vi "FindBandwidth.vi"() -> ()   [LabVIEW 2022 SP3]
doc: "6/7/11- It doesnt really work."
uses:
  <vilib>/Analysis/baseanly.llb/Mean (DBL).vi
  <vilib>/Utility/file.llb/Read Delimited Spreadsheet (DBL).vi
  <vilib>/Analysis/NI_AALBase.lvlib
panel:
  in  "Define BW?":bool
  in  "non dB data?":bool=TRUE
  out "Array 2":T1(array[cluster]) {"bandwidth" format="%.2f"; "upper band freq" format="%.2f"; "lower band freq" format="%.2f"; "center freq" format="%.2f"; "max freq (dB)" format="%.2f"; "max f" format="%.2f"}
  out "DOF":cluster{dbl[], sgl[]}(graph)
  out "L BW":cluster{dbl[], dbl[]}(graph)
  in  "f cut off MHz":dbl=100.0
  out "Array":dbl[][](array[numeric])
  in  "file ext":string="*.txt"
  in  "Use Selected Files":bool
  in  "Listbox":i32[](listbox)
  in  "Choose Directory":path
  in  "Save path":path
  in  "Save?":bool
  out "XY Graph":cluster{"all rows":dbl[], "all rows":dbl[]}[](graph)
  in  "Save spectrum only":bool
  in  "dB width pt":dbl=-6.0 format="%.2f"
  # "max f"
  # "max f dB"
  # "fc 15 dB"
  # "BW 15db"
  # "fc 6 db"
  # "BW 6dB"
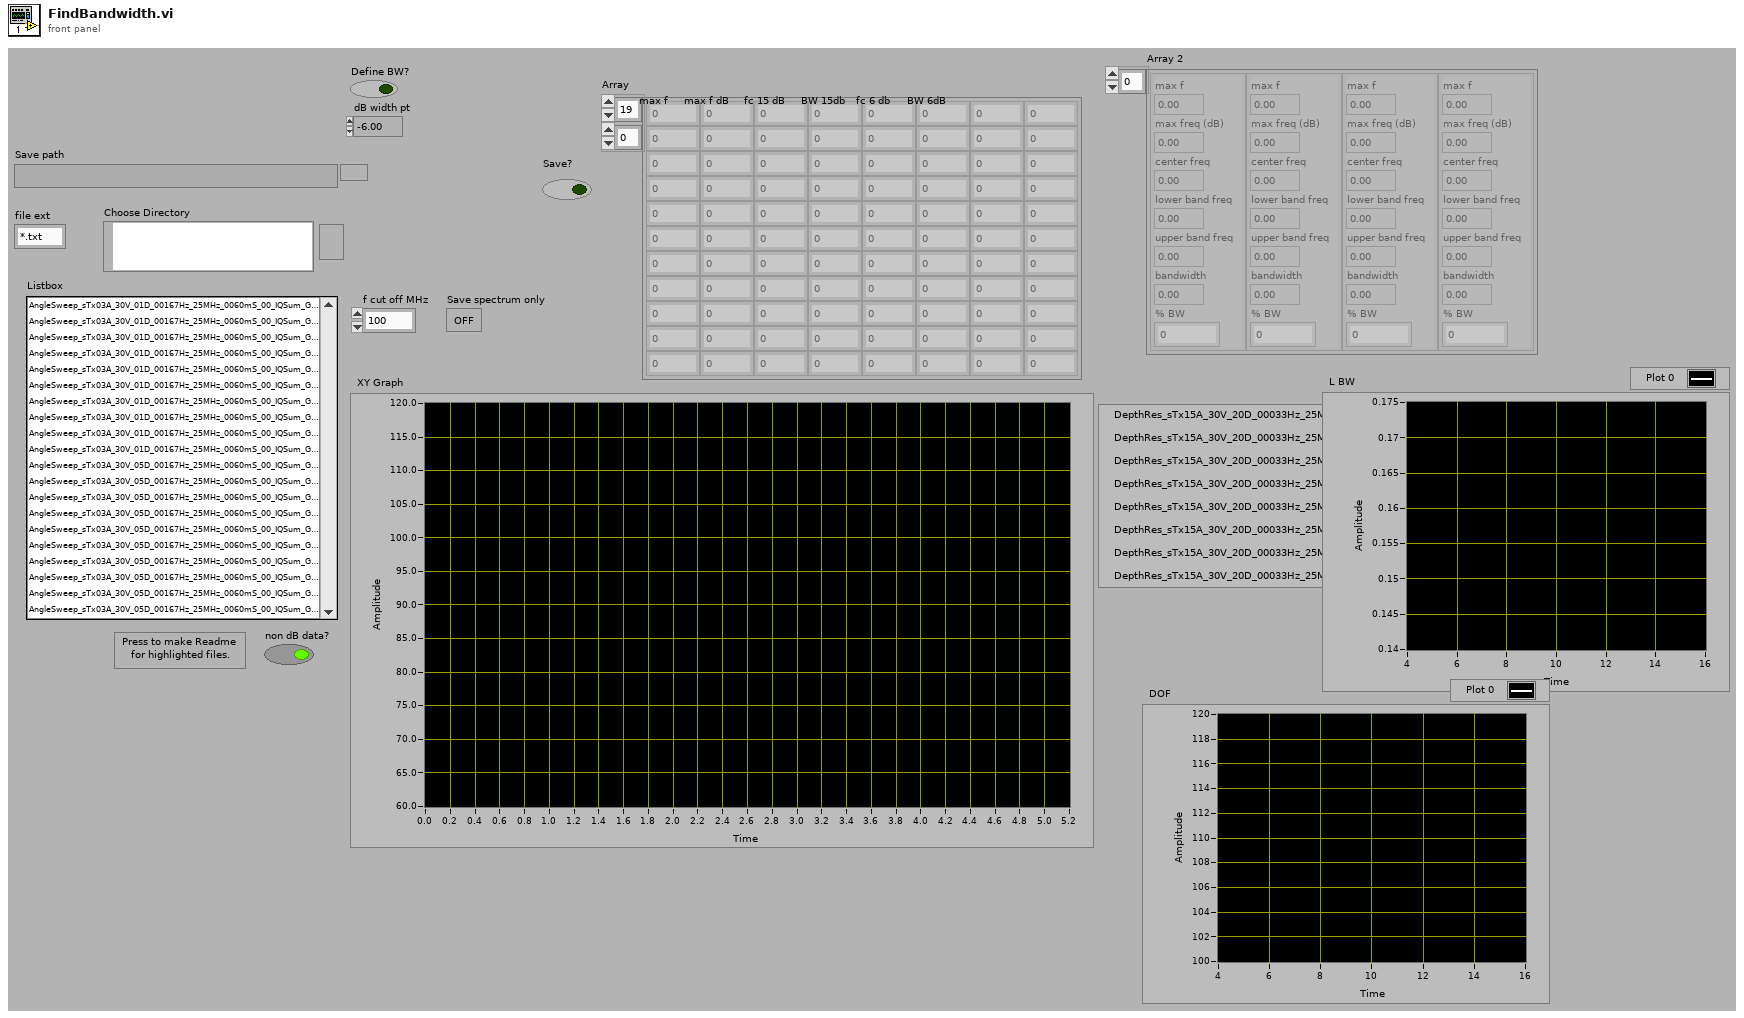
[diagram p1: front panel]
types:
  T1 = cluster{"max f":sgl, "max freq (dB)":sgl, "center freq":sgl, "lower band freq":sgl, "upper band freq":sgl, "bandwidth":sgl, "% BW":dbl}[]
  T2 = cluster{"max f":sgl, "max freq (dB)":sgl, "center freq":sgl, "lower band freq":sgl, "upper band freq":sgl, "bandwidth":sgl, "% BW":dbl}
  T3 = enum16{"open", "replace", "create", "open or create", "replace or create", "replace or create with confirmation"}
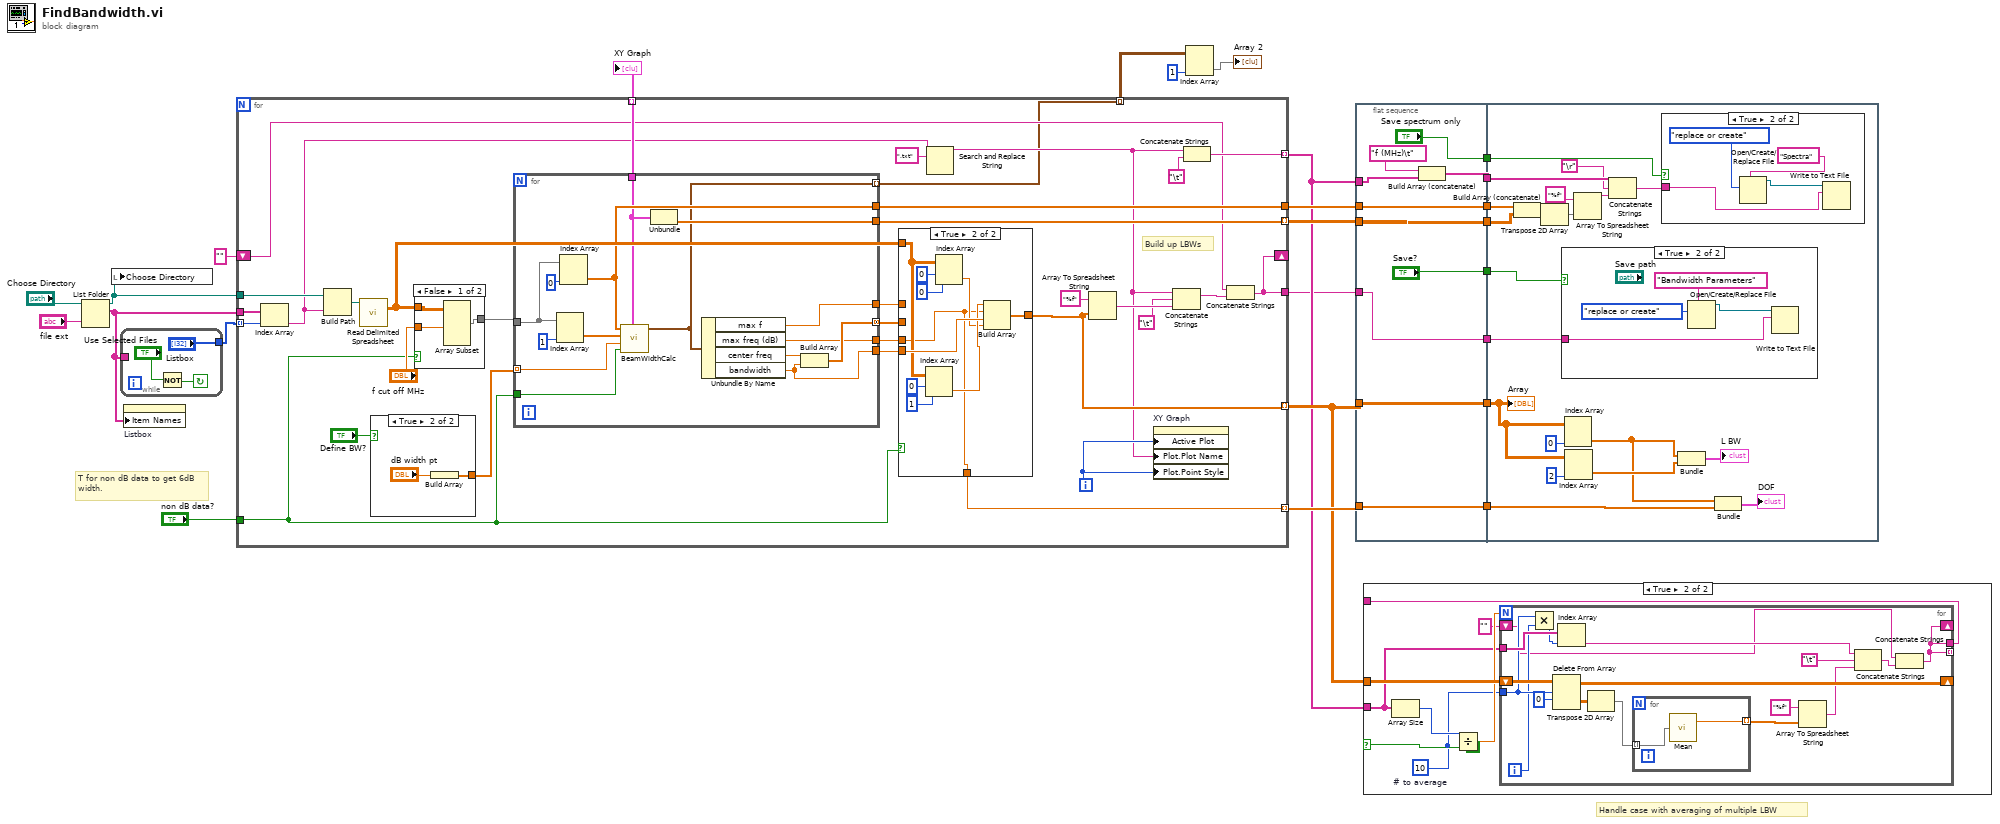
[diagram p0: block diagram]
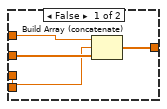
[diagram p5: hidden frame]
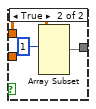
[diagram p6: hidden frame]
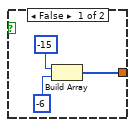
[diagram p7: hidden frame]
diagram:
  # "Handle case with averaging of multiple LBW"
  # "T for non dB data to get 6dB width."
  n1 = List Folder(path="Choose Directory", pattern="file ext") -> (path out=w24:path, filenames=w23:string[])  [unwired: 1 in, 3 out]
  n2 = local write "Choose Directory"(w24) -> ()
  n3 = while {
    tunnel: ["Listbox"] -> w6
    tunnel: w23 -> [_]
    stop <- w29 continue-if-true
    n4 = Not(x="Use Selected Files") -> (.not. x?=w29:bool)
  }
  n5 = property on="Listbox" class="LstBox (strict)"("Item Names"=w23) -> ()  [unwired: 2 in, 2 out]
  n6 = for {
    tunnel: w24 -> [w60]
    tunnel: w23 -> [w58]
    tunnel: w6 -> [w32] mode=indexing
    tunnel: [w53] -> w5 mode=indexing
    tunnel: [w57] -> w22 mode=indexing
    tunnel: [w52] -> w21 mode=indexing
    tunnel: [w51] -> w20
    tunnel: [w30] -> w2
    tunnel: [w47] -> w4 mode=indexing
    shift-right: [w30] -> _
    shift-left: "" -> [w43]
    tunnel: "non dB data?" -> [w37]
    tunnel: [w35] -> w10 mode=indexing
    tunnel: [w33] -> w9 mode=indexing
    i -> [w49]
    # "Build up LBWs"
    n7 = Index Array(array=w58, index=w32) -> (element=w46:string)
    n8 = Build Path(base path=w60, name or relative path=w46) -> (appended path=w59:path)
    n9 = call-poly <vilib>:"Read Delimited Spreadsheet.vi"("file path (dialog if empty)"=w59) -> ("all rows"=w38:dbl[][])  [unwired: 9 in, 5 out]
    n10 = case shown="True" "Define BW?" {
      tunnel: [w82 w85] -> w61
      frame False {
        n11 = Build Array(-15, -6) -> (w82:i32[])
      }
      frame True {
        n12 = Build Array("dB width pt") -> (w85:dbl[])
      }
    }
    n13 = case shown="False" w37 {
      tunnel: [w76 w81] -> w42
      tunnel: w38 -> [w78 w79]
      tunnel: "f cut off MHz" -> [w77 _]
      frame False {
        n14 = Array Subset(array=w78, length (row)=w77) -> (w76:dbl[][])  [unwired: 3 in]
      }
      frame True {
        n15 = Array Subset(array=w79, index (row)=1 ("index")) -> (w81:dbl[][])  [unwired: 3 in]
      }
    }
    n16 = for {
      tunnel: w61 -> [w99] mode=indexing
      tunnel: [w94] -> w36
      tunnel: [w92] -> w41
      tunnel: [w89] -> w57
      tunnel: [w88] -> w52
      tunnel: [w97] -> w51
      tunnel: w42 -> [w98]
      tunnel: [w96] -> w39 mode=concatenating
      tunnel: w37 -> [w91]
      tunnel: [w93] -> w34
      tunnel: [w87] -> w33 mode=indexing
      n17 = Index Array(array=w98, index (col)=1) -> (element=w90:dbl[])  [unwired: 1 in]
      n18 = Index Array(array=w98, index (col)=0) -> (element=w97:dbl[])  [unwired: 1 in]
      n19 = call "BeamWidthCalc.vi"("Not dB?"=w91, "dB width pt"=w99, "y values"=w90, "x values"=w97) -> ("Output variables"=w87:T2, "Plot Values"=w89:cluster{dbl[], dbl[]})  [unwired: 5 in, 1 out]
      n20 = Unbundle(w89) -> (w88:dbl[])  [unwired: 1 out]
      n21 = Unbundle By Name(w87) -> ("max f"=w94:sgl, "max freq (dB)"=w93:sgl, "center freq"=w95:sgl, "bandwidth"=w92:sgl)
      n22 = Build Array(w95, w92) -> (w96:sgl[])
    }
    n23 = case shown="True" w37 {
      tunnel: w34 -> [w62 w66]
      tunnel: [w64 w75] -> w53
      tunnel: w38 -> [_ w68]
      tunnel: w41 -> [_ w74]
      tunnel: w39 -> [w65 _]
      tunnel: w36 -> [w63 _]
      tunnel: [_ w66] -> w35
      frame False {
        n24 = Build Array (concatenate)(w63, w62, w65) -> (w64:sgl[])
      }
      frame True {
        n25 = Index Array(array=w68, index (row)=0, index (col)=1 ("disabled index (col)")) -> (element=w69:dbl)
        n26 = Index Array(array=w68, index (row)=0, index (col)=0 ("disabled index (col)")) -> (element=w67:dbl)
        n27 = Build Array(w69, w66, w74, w67) -> (w75:dbl[])
      }
    }
    n28 = Search and Replace String(input string=w46, search string=".txt") -> (result string=w44:string)  [unwired: 6 in, 3 out]
    n29 = Array To Spreadsheet String(array=w53, 3:"%f" ("format string")) -> (spreadsheet string=w56:string)  [unwired: 1 in]
    n30 = property on="XY Graph" class="XYGraph (strict)"("Active Plot"=w49, "Plot.Plot Name"=w44, "Plot.Point Style"=w49) -> ()  [unwired: 2 in, 2 out]
    n31 = Concatenate Strings(w44, "\t", w56) -> (w50:string)
    n32 = Concatenate Strings(w44, "\t") -> (w47:string)
    n33 = Concatenate Strings(w43, w50) -> (w30:string)
  }
  "XY Graph" <- w22
  n34 = Index Array(array=w9, index (col)=1 ("disabled index (col)")) -> (element=→"Array 2":T1)  [unwired: 1 in]
  n35 = flat-sequence {
    tunnel: w20 -> [w109]
    tunnel: w21 -> [w110]
    tunnel: w5 -> [w111]
    tunnel: [w111] -> w19
    tunnel: ["Save?"] -> w18
    tunnel: [w110] -> w17
    tunnel: [w109] -> w16
    tunnel: ["Save spectrum only"] -> w15
    tunnel: w2 -> [w106]
    tunnel: [w106] -> w14
    tunnel: [w105] -> w13
    tunnel: w4 -> [w103]
    tunnel: [w102] -> w11
    tunnel: w10 -> [w102]
    tunnel: w19 -> [w112]
    tunnel: w18 -> [w131]
    tunnel: w17 -> [w130]
    tunnel: w16 -> [w129]
    tunnel: w15 -> [w128]
    tunnel: w14 -> [w127]
    tunnel: w13 -> [w121]
    tunnel: w11 -> [w114]
    frame #0 {
      n36 = Build Array (concatenate)("f (MHz)\t", w103) -> (w105:string[])
    }
    frame #1 {
      n37 = Build Array (concatenate)(w129, w130) -> (w126:dbl[][])
      n38 = Transpose 2D Array(2D array=w126) -> (transposed array=w122:dbl[][])
      n39 = case shown="True" w131 {
        tunnel: w127 -> [_ w139]
        frame False {
        }
        frame True {
          n40 = Open/Create/Replace File(prompt="Bandwidth Parameters", operation (0:open)=T3."replace or create") -> (refnum out=w138:refnum<file>)  [unwired: 4 in, 2 out]
          n41 = Write to Text File(file (use dialog)=w138, text=w139) -> ()  [unwired: 2 in, 3 out]
        }
      }
      n42 = Index Array(array=w112, index (col)=0 ("disabled index (col)")) -> (element=w113:dbl[])  [unwired: 1 in]
      n43 = Index Array(array=w112, index (col)=2 ("disabled index (col)")) -> (element=w117:dbl[])  [unwired: 1 in]
      n44 = Array To Spreadsheet String(array=w122, 3:"%f" ("format string")) -> (spreadsheet string=w124:string)  [unwired: 1 in]
      n45 = Concatenate Strings(w121, "\r", w124) -> (w123:string)
      n46 = case shown="True" w128 {
        tunnel: w123 -> [_ w133]
        frame False {
        }
        frame True {
          n47 = Open/Create/Replace File(prompt="Spectra", operation (0:open)=T3."replace or create") -> (refnum out=w135:refnum<file>)  [unwired: 4 in, 2 out]
          n48 = Write to Text File(file (use dialog)=w135, text=w133) -> ()  [unwired: 2 in, 3 out]
        }
      }
      n49 = Bundle(w113, w117) -> (→"L BW":cluster{dbl[], dbl[]})  [unwired: 1 in]
      n50 = Bundle(w113, w114) -> (→"DOF":cluster{dbl[], sgl[]})  [unwired: 1 in]
      "Array" <- w112
    }
  }
  n51 = case shown="True" FALSE {
    tunnel: w5 -> [_ w145]
    tunnel: w4 -> [_ w140]
    tunnel: [_ w142] -> _
    frame False {
    }
    frame True {
      w143 = 10  # # to average
      n52 = Array Size(array=w140) -> (size(s)=w146:i32)
      n53 = Divide(x=w146, y=w143) -> (x/y=w144:dbl)
      n54 = for {
        N: w144 -> [_]
        shift-right: [w162] -> _
        shift-left: w145 -> [w163]
        tunnel: w143 -> [w157]
        tunnel: w140 -> [w158]
        tunnel: [w147] -> w142
        shift-right: [w147] -> _
        shift-left: "" -> [w148]
        tunnel: [w147] -> _ mode=indexing
        i -> [w156]
        n55 = Multiply(x=w157, y=w156) -> (x*y=w155:i32)
        n56 = Delete From Array(array=w163, length=w157, index (row)=0) -> (deleted portion=w161:dbl[][], array with subset deleted=w162:dbl[][])  [unwired: 1 in]
        n57 = Index Array(array=w158, index=w155) -> (element=w150:string)
        n58 = Transpose 2D Array(2D array=w161) -> (transposed array=w160:dbl[][])
        n59 = for {
          tunnel: w160 -> [w165] mode=indexing
          tunnel: [w164] -> w151 mode=indexing
          n60 = call-poly <vilib>:"Mean.vi"("X"=w165) -> ("mean"=w164:dbl)  [unwired: 1 out]
        }
        n61 = Array To Spreadsheet String(array=w151, 3:"%f" ("format string")) -> (spreadsheet string=w154:string)  [unwired: 1 in]
        n62 = Concatenate Strings(w150, "\t", w154) -> (w149:string)
        n63 = Concatenate Strings(w148, w149) -> (w147:string)
      }
    }
  }
